vi "GTH-V2.Relays.vi"(7 "CMD":enum16{"All", "ChanA", "ChanB", "Single"}(ring), 8 "Error In":errorcluster caption="错误输入", 9 "ON/FF":bool, 10 "Para":T1(ring), 11 "VISA资源输入":refnum<visa-resource-name>) -> (0 "Error Out":errorcluster caption="错误输出", 2 "命令":string, 3 "OK?":bool)   [LabVIEW 2012, in "Lib_UEL.ATE.lvlib" / "STM32-CoreBD.lvlib"]
uses:
  STM32-CoreBD.lvlib
panel:
  # "Version History\nV1.0.0,2015-8-4, 适用于新版GTH-V2硬件."
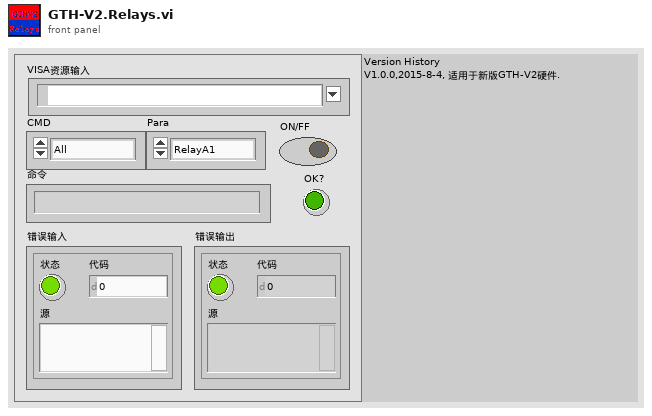
[diagram p1: front panel]
types:
  T1 = enum16{"RelayA1", "RelayA2", "RelayA3", "RelayA4", "RelayA5", "RelayA6", "RelayA7", "RelayA8", "RelayA9", "RelayA10", "RelayB1", "RelayB2", "RelayB3", "RelayB4", "RelayB5", "RelayB6", "RelayB7", "RelayB8", "RelayB9", "RelayB10", "ADC1", "ADC2", "ADC3", "DAC1"}
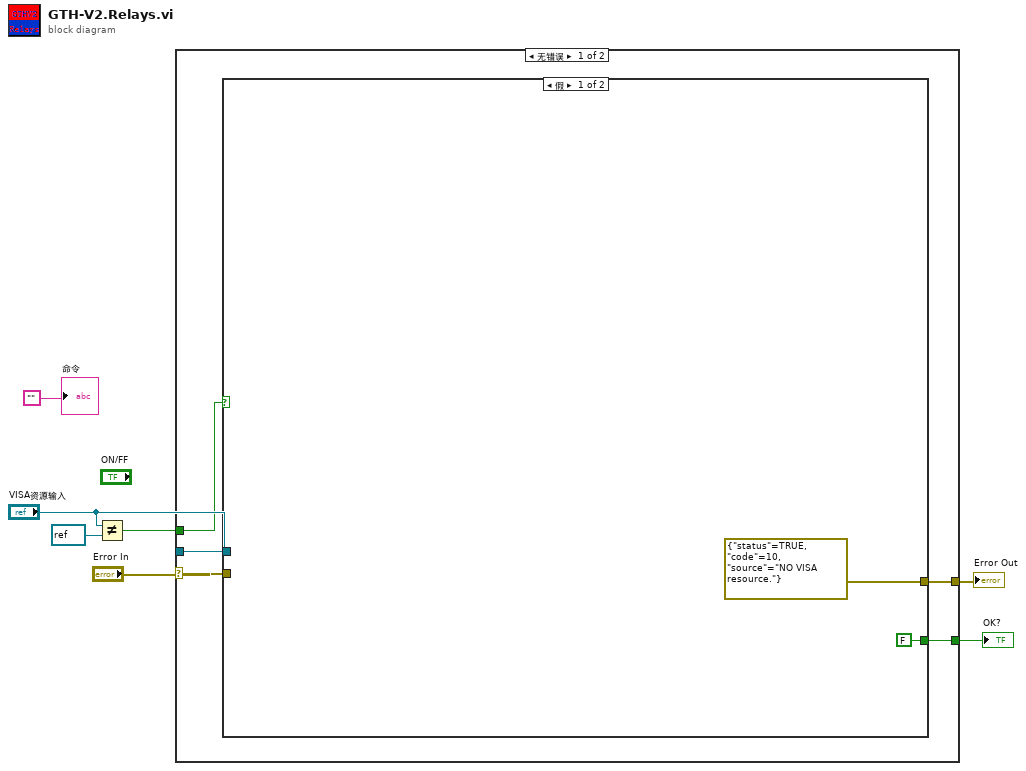
[diagram p0: block diagram]
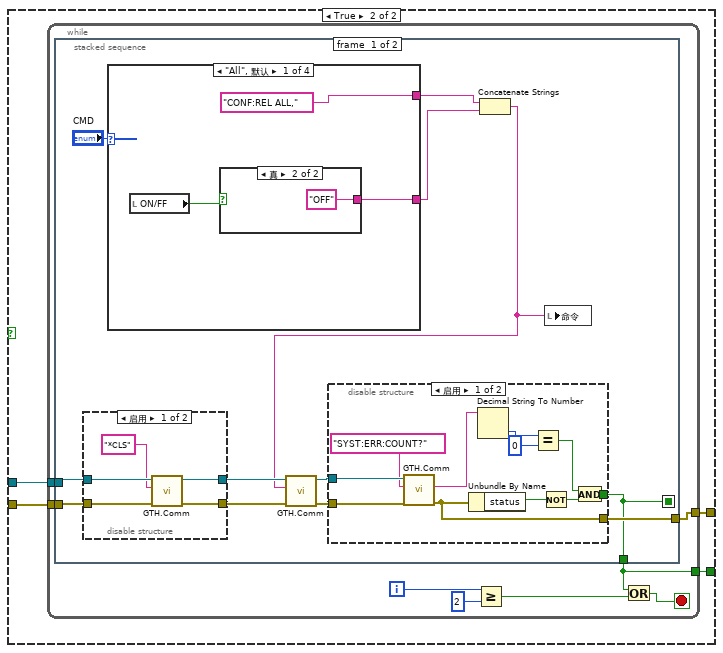
[diagram p2: hidden frame]
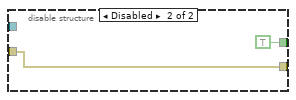
[diagram p3: hidden frame]
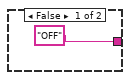
[diagram p5: hidden frame]
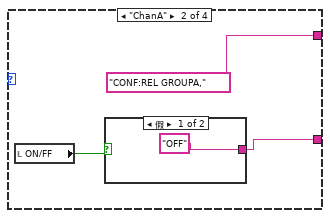
[diagram p6: hidden frame]
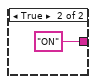
[diagram p7: hidden frame]
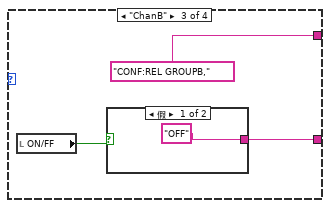
[diagram p8: hidden frame]
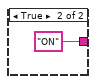
[diagram p9: hidden frame]
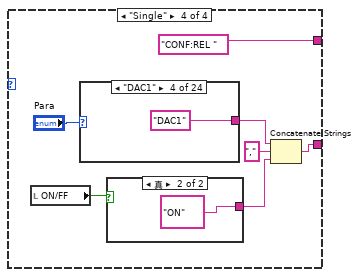
[diagram p10: hidden frame]
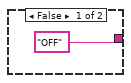
[diagram p11: hidden frame]
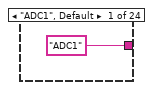
[diagram p12: hidden frame]
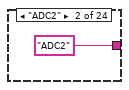
[diagram p13: hidden frame]
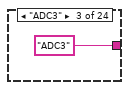
[diagram p14: hidden frame]
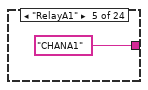
[diagram p15: hidden frame]
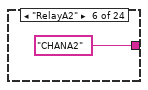
[diagram p16: hidden frame]
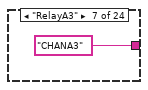
[diagram p17: hidden frame]
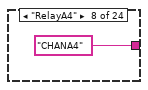
[diagram p18: hidden frame]
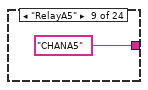
[diagram p19: hidden frame]
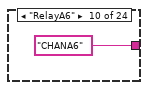
[diagram p20: hidden frame]
diagram:
  n1 = Not Equal?(x="VISA资源输入", y=refnum<visa-resource-name> refnum) -> (x != y?=w1:bool)
  n2 = case shown="无错误" "Error In" {
    selector: "Error In" -> [w11 w110]
    tunnel: [w10 w110] -> w7
    tunnel: "VISA资源输入" -> [w12 _]
    tunnel: [w9 FALSE] -> w4
    tunnel: w1 -> [w8 _]
    frame No Error {
      n3 = case shown="假" w8 {
        tunnel: w12 -> [_ w18]
        tunnel: w11 -> [_ w17]
        tunnel: [errorcluster {"status"=TRUE, "code"=10, "source"="NO VISA resource."} ("Error Out") w16] -> w10
        tunnel: [FALSE w15] -> w9
        frame False {
        }
        frame True {
          n4 = while {
            tunnel: w18 -> [w26]
            tunnel: w17 -> [w25]
            tunnel: [w24] -> w16
            tunnel: [w19] -> w15
            i -> [w22]
            stop <- w23 stop-if-true
            n5 = stacked-sequence {
              seq-local: [w27 _] -> [_ w107]
              tunnel: w26 -> [w36 _]
              tunnel: w25 -> [w35 _]
              tunnel: [w28 _] -> w24
              tunnel: [w27 _] -> w19
              frame #0 {
                n6 = disable-structure shown="启用" {
                  disable-tunnel: w36 -> [w56 w58]
                  disable-tunnel: w35 -> [w55 w57]
                  disable-tunnel: [w53 w58] -> w34
                  disable-tunnel: [w52 w57] -> w33
                  frame Enabled {
                    n7 = call "GTH.Comm.vi"("Error In"=w55, "SCPI CMD"="*CLS", "USB Port In"=w56) -> ("Error Out"=w52:errorcluster, "USB Port Out"=w53:refnum<visa-resource-name>)  [unwired: 3 in, 4 out]
                  }
                  frame Disabled {
                  }
                }
                n8 = case shown="\"All\", 默认" "CMD" {
                  tunnel: ["CONF:REL ALL," ("字符串") "CONF:REL GROUPA," ("字符串") "CONF:REL GROUPB," ("字符串") "CONF:REL " ("字符串")] -> w32
                  tunnel: [w60 w64 w69 w77] -> w37
                  frame "All", Default {
                    n9 = local read "ON/FF"() -> (w59:bool)
                    n10 = case shown="真" w59 {
                      tunnel: ["OFF" ("字符串") "OFF" ("字符串")] -> w60
                      frame False {
                      }
                      frame True {
                      }
                    }
                  }
                  frame "ChanA" {
                    n11 = local read "ON/FF"() -> (w65:bool)
                    n12 = case shown="假" w65 {
                      tunnel: ["OFF" ("字符串") "ON" ("字符串")] -> w64
                      frame False {
                      }
                      frame True {
                      }
                    }
                  }
                  frame "ChanB" {
                    n13 = local read "ON/FF"() -> (w70:bool)
                    n14 = case shown="假" w70 {
                      tunnel: ["OFF" ("字符串") "ON" ("字符串")] -> w69
                      frame False {
                      }
                      frame True {
                      }
                    }
                  }
                  frame "Single" {
                    n15 = local read "ON/FF"() -> (w78:bool)
                    n16 = case shown="\"DAC1\"" "Para" {
                      tunnel: ["ADC1" ("字符串") "ADC2" ("字符串") "ADC3" ("字符串") "DAC1" ("字符串") "CHANA1" ("字符串") "CHANA2" ("字符串") "CHANA3" ("字符串") "CHANA4" ("字符串") "CHANA5" ("字符串") "CHANA6" ("字符串") "CHANA7" ("字符串") "CHANA8" ("字符串") "CHANA9" ("字符串") "CHANA10" ("字符串") "CHANB1" ("字符串") "CHANB2" ("字符串") "CHANB3" ("字符串") "CHANB4" ("字符串") "CHANB5" ("字符串") "CHANB6" ("字符串") "CHANB7" ("字符串") "CHANB8" ("字符串") "CHANB9" ("字符串") "CHANB10" ("字符串")] -> w76
                      frame "ADC1", Default {
                      }
                      frame "ADC2" {
                      }
                      frame "ADC3" {
                      }
                      frame "DAC1" {
                      }
                      frame "RelayA1" {
                      }
                      frame "RelayA2" {
                      }
                      frame "RelayA3" {
                      }
                      frame "RelayA4" {
                      }
                      frame "RelayA5" {
                      }
                      frame "RelayA6" {
                      }
                      frame "RelayA7" {
                      }
                      frame "RelayA8" {
                      }
                      frame "RelayA9" {
                      }
                      frame "RelayA10" {
                      }
                      frame "RelayB1" {
                      }
                      frame "RelayB2" {
                      }
                      frame "RelayB3" {
                      }
                      frame "RelayB4" {
                      }
                      frame "RelayB5" {
                      }
                      frame "RelayB6" {
                      }
                      frame "RelayB7" {
                      }
                      frame "RelayB8" {
                      }
                      frame "RelayB9" {
                      }
                      frame "RelayB10" {
                      }
                    }
                    n17 = case shown="真" w78 {
                      tunnel: ["OFF" ("字符串") "ON" ("字符串")] -> w75
                      frame False {
                      }
                      frame True {
                      }
                    }
                    n18 = Concatenate Strings(w76, "," ("字符串"), w75) -> (w77:string)
                  }
                }
                n19 = Concatenate Strings(w32, w37) -> (w31:string)
                n20 = call "GTH.Comm.vi"("Error In"=w33, "SCPI CMD"=w31, "USB Port In"=w34) -> ("Error Out"=w29:errorcluster, "USB Port Out"=w30:refnum<visa-resource-name>)  [unwired: 3 in, 4 out]
                n21 = disable-structure shown="启用" {
                  disable-tunnel: w30 -> [w49 _]
                  disable-tunnel: w29 -> [w48 w51]
                  disable-tunnel: [w43 w51] -> w28
                  disable-tunnel: [w39 TRUE] -> w27
                  frame Enabled {
                    n22 = call "GTH.Comm.vi"("Error In"=w48, "SCPI CMD"="SYST:ERR:COUNT?", "USB Port In"=w49) -> ("Error Out"=w43:errorcluster, "Return"=w46:string)  [unwired: 3 in, 4 out]
                    n23 = Unbundle By Name(w43) -> ("status"=w42:bool)
                    n24 = Decimal String To Number(string=w46) -> (number=w45:i32)  [unwired: 2 in, 1 out]
                    n25 = Equal?(x=w45, y=0) -> (x = y?=w40:bool)
                    n26 = Not(x=w42) -> (.not. x?=w41:bool)
                    n27 = And(x=w40, y=w41) -> (x .and. y?=w39:bool)
                  }
                  frame Disabled {
                  }
                }
                n28 = local write "命令"(w31) -> ()
              }
              frame #1 {
                n29 = case shown="假" w107 {
                  frame False {
                    n30 = Wait (ms)(milliseconds to wait=u32 800 ("等待时间（毫秒）")) -> ()  [unwired: 1 out]
                  }
                  frame True {
                  }
                }
              }
            }
            n31 = Greater Or Equal?(x=w22, y=2) -> (x >= y?=w20:bool)
            n32 = Or(x=w19, y=w20) -> (x .or. y?=w23:bool)
          }
        }
      }
    }
    frame Error {
    }
  }
  "Error Out" <- w7
  "OK?" <- w4
  "命令" <- ""
